vi "Pointer.Duration.vi"() -> ()   [LabVIEW 2016]
uses:
  <vilib>/Platform/TimedLoop/XDataNode/timing_clust.ctl
  <vilib>/Platform/TimedLoop/XDataNode/nitl_modes.ctl
  <vilib>/Platform/TimedLoop/XDataNode/wakeup.ctl
  Library/Classes/Pointer/Memory.Pointer.lvclass/Memory.Pointer.ctl
  Library/Classes/Pointer/Methods/Memory.Pointer.Read.All.In Place.Unsafe (1D U8).vi
  Library/Classes/Pointer/Methods/Accessors/Memory.Pointer.Get Address.vi
  Library/Classes/Pointer/Methods/Accessors/Memory.Pointer.Get Size.vi
  Library/Classes/Pointer/Methods/Memory.Pointer.Allocate.vi
  Library/Classes/Pointer/Methods/Accessors/Memory.Pointer.Set Address.vi
  Library/Classes/Pointer/Methods/Accessors/Memory.Pointer.Set Size.vi
  Library/Classes/Pointer/Methods/Memory.Pointer.Bounds Check.Size.vi
  <vilib>/platform/TimedLoop/XDataNode/XDataNode.xnode
  Library/Classes/Pointer/Memory.Pointer.lvclass
  <vilib>/Platform/TimedLoop/XDataNode/XDNodeRunTimeDep.lvlib
panel:
  out "Numeric":u32
  out "avg duration":dbl format="%.3ps"
  in  "iterations":i32=10000000 format="%.0p"
  in  "processor":i32=-2
  in  "size":i64=1024 format="%d bytes"
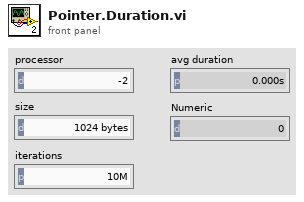
[diagram p1: front panel]
types:
  T1 = typedef "XDNodeRunTimeDep.lvlib/timing_clust.ctl" = cluster{"Expected End [f-1]":u64, "Actual End [f-1]":u64, "Finished Late? [f-1]":bool, "Expected End [i-1]":u64, "Actual End [i-1]":u64, "Finished Late? [i-1]":bool, "Expected Start [i]":u64, "Actual Start [i]":u64, "Expected Start [f]":u64, "Actual Start [f]":u64, "Source Name":string, "Structure Name":string, "Period":i64, "Deadline":i64, "Offset":i64, "Start":i64, "Priority":i32, "Timeout":i32, "Mode":T2, "Wakeup Reason":T3, "Error":errorcluster, "Source Type":string, "Secondary Source Type":string, "Global End Time":u64, "Global Start Time":u64, "Frame Duration":u64, "Iteration Duration":u64, "Assigned CPU":i32, "I/O Scan Engine Mode":u32}
  T2 = typedef "XDNodeRunTimeDep.lvlib/nitl_modes.ctl" = enum32{"No Change", "Process missed periods, maintain original phase", "Discard missed periods, maintain original phase", "Process missed periods, ignore original phase", "Discard missed periods, ignore original phase"}
  T3 = typedef "XDNodeRunTimeDep.lvlib/wakeup.ctl" = enum32{"Normal", "Aborted", "Asynchronous wakeup", "Timing source error", "Timed loop error", "Timeout"}
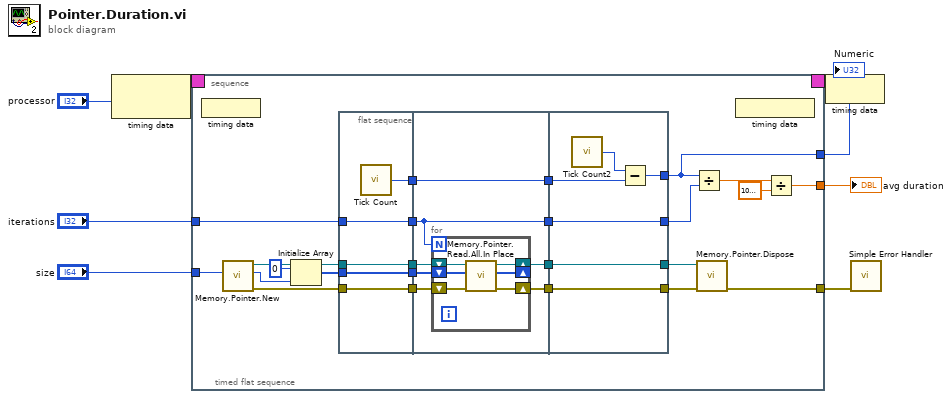
[diagram p0: block diagram]
diagram:
  n1 = node-c288("processor") -> (w8:T1)
  n2 = timed-sequence {
    timing: w8 -> [_]
    timing-out: [_] -> w7
    tunnel: "iterations" -> [w13]
    tunnel: "size" -> [w12]
    tunnel: [w11] -> w3
    tunnel: [w10] -> w2
    tunnel: [w9] -> w1
    n3 = timed-flat-sequence {
      tunnel: w13 -> [w36]
      tunnel: w12 -> [w22]
      tunnel: [w19] -> w11
      tunnel: [w17] -> w10
      tunnel: [w14] -> w9
      n4 = node-c288() -> ()  [unwired: 1 in]
      n5 = call "Memory.Pointer.New.vi"("size"=w22) -> ("error out"=w28:errorcluster, "allocated size"=w23:i64, "Pointer out"=w29:refnum<class "Memory.Pointer.lvclass">)  [unwired: 8 in]
      n6 = Initialize Array(u8 0 ("element"), w23) -> (w16:u8[])
      n7 = flat-sequence {
        tunnel: [w42] -> w35
        tunnel: [w41] -> w34
        tunnel: [w40] -> w30
        tunnel: [w39] -> w27
        tunnel: [w38] -> w24
        tunnel: w36 -> [w42]
        tunnel: w29 -> [w40]
        tunnel: w28 -> [w39]
        tunnel: w16 -> [w38]
        tunnel: w35 -> [w48]
        tunnel: w34 -> [w49]
        tunnel: [w49] -> w33
        tunnel: [w48] -> w32
        tunnel: w30 -> [w47]
        tunnel: w27 -> [w46]
        tunnel: [w45] -> w26
        tunnel: [w44] -> w25
        tunnel: w24 -> [w43]
        tunnel: w33 -> [w60]
        tunnel: w32 -> [w59]
        tunnel: [w59] -> w37
        tunnel: [w58] -> w14
        tunnel: w26 -> [w57]
        tunnel: [w57] -> w21
        tunnel: w25 -> [w56]
        tunnel: [w56] -> w20
        frame #0 {
          n8 = call "Tick Count"() -> ("Tick Count(uSec)"=w41:u32)
        }
        frame #1 {
          n9 = for {
            N: w48 -> [_]
            shift-right: [w53] -> w44
            shift-left: w47 -> [w55]
            shift-right: [w52] -> _
            shift-left: w43 -> [w54]
            shift-right: [w51] -> w45
            shift-left: w46 -> [w50]
            n10 = call-poly "Memory.Pointer.Read.All.In Place.vi"("error in (no error)"=w50, "buffer in"=w54, "Pointer in"=w55) -> ("error out"=w51:errorcluster, "buffer out"=w52:u8[], "Pointer out"=w53:refnum<class "Memory.Pointer.lvclass">)  [unwired: 6 in]
          }
        }
        frame #2 {
          n11 = call "Tick Count2"() -> ("Tick Count(uSec)"=w61:u32)
          n12 = Subtract(x=w61, y=w60) -> (x-y=w58:u32)
        }
      }
      n13 = Divide(x=w14, y=w37) -> (x/y=w15:dbl)
      n14 = call "Memory.Pointer.Dispose.vi"("error in (no error)"=w21, "Pointer in"=w20) -> ("error out"=w19:errorcluster)  [unwired: 9 in]
      n15 = node-c288() -> ()  [unwired: 1 out]
      n16 = Divide(x=w15, y=1000000.0) -> (x/y=w17:dbl)
    }
  }
  "avg duration" <- w2
  "Numeric" <- w1
  n17 = node-c288(w7) -> ()
  n18 = call <vilib>:"Simple Error Handler.vi"("error in (no error)"=w3) -> ()  [unwired: 4 in, 5 out]
